vi "SetScanDataGetStatusToYes.vi"(8 "error in (no error)":errorcluster, 9 "Yes?":bool=TRUE, 10 "Device Name":string, 11 "Experiment Name":string) -> (0 "error out":errorcluster)   [LabVIEW 2020]
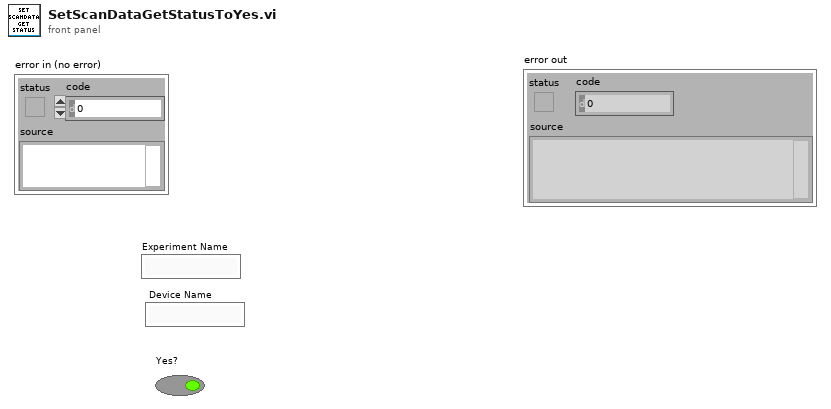
[diagram p1: front panel]
types:
  T1 = typedef "mysql_authentication.ctl" = cluster{"User":string, "Password":string, "Database":string}
  T2 = cluster{"Port":u16, "IP Address":string, "Authentication":T1}
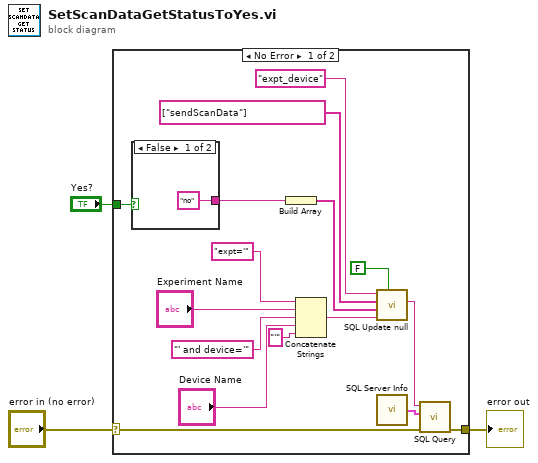
[diagram p0: block diagram]
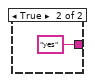
[diagram p2: hidden frame]
diagram:
  n1 = case shown="No Error" "error in (no error)" {
    selector: "error in (no error)" -> [w6 w22]
    tunnel: [w10 w22] -> w3
    tunnel: "Yes?" -> [w4 _]
    frame No Error {
      n2 = case shown="False" w4 {
        tunnel: ["no" ("Table") "yes" ("Table")] -> w5
        frame False {
        }
        frame True {
        }
      }
      n3 = Build Array(w5) -> (w15:string[])
      n4 = Concatenate Strings("expt='", "Experiment Name", "' and device='" ("string"), "Device Name", "'" ("string")) -> (w12:string)
      n5 = call "SQL Update null.vi"("Use Empty String as Ignore? (T)"=FALSE, "Where clause"=w12, "Values"=w15, "Column Names"=string[] ["sendScanData"], "Table"="expt_device") -> ("Query String"=w17:string)  [unwired: 6 in]
      n6 = call "SQL Server Info.vi"() -> ("SQL Server Info"=w16:T2)
      n7 = call "SQL Query.vi"("error in (no error)"=w6, "SQL Server Info"=w16, "Query"=w17) -> ("error out"=w10:errorcluster)  [unwired: 7 in, 1 out]
    }
    frame Error {
    }
  }
  "error out" <- w3
